vi "Get Analog Replay Settings.vi"(8 "error in (no error)":errorcluster, 11 "Analog Replay in":refnum<k24>) -> (0 "error out":errorcluster, 1 "Analog Replay Data Options":T1={"Input file"=path "", "Group"="", "Channel"="", "Reverse"=FALSE, "FPGA Memory Size"=enum."16,384", "Position reference"=enum."Crank angle", "Data selection method"=enum."Manual", "Offset"=0, "Samples"=0, "Missing teeth location"=0.0, "DataPlugin"=""}, 2 "Analog Replay Settings":T5={"Name"="", "DAC bipolar range (V)"=0.0, "Voltage below min speed"=0.0, "Min speed (RPM)"=0.0, "Voltage at min speed"=0.0, "Max speed (RPM)"=0.0, "Voltage at max speed"=0.0, "Negate playback voltage values at negative engine speed"=TRUE, "Allow run-time override of voltage scaling"=FALSE}, 3 "Analog Replay out":refnum<k24>)   [LabVIEW 2015, in "Engine Simulation Toolkit SysDef API.lvlib"]
uses:
  Engine Simulation Toolkit SysDef API.lvlib
  NationalInstruments.VeriStand.SystemDefinitionAPI
  Analog Replay Settings.ctl
  Analog Replay Data Options.ctl
  System Explorer/FPGA Mem Size.ctl
  System Explorer/Position Reference.ctl
  System Explorer/Data Replay Data Selection Method.ctl
  Shared/Properties.vi
  <vilib>/NI Veristand/Custom Device API/Get Item Property (String).vi
  <vilib>/NI Veristand/Custom Device API/Get Item Property (Double).vi
  <vilib>/NI Veristand/Custom Device API/Get Item Property (Boolean).vi
  Shared/Engine Simulation Toolkit Shared.lvlib
  System Explorer/Engine Simulation Toolkit System Explorer.lvlib
  <vilib>/NI VeriStand/Custom Device API/Custom Device API.lvlib
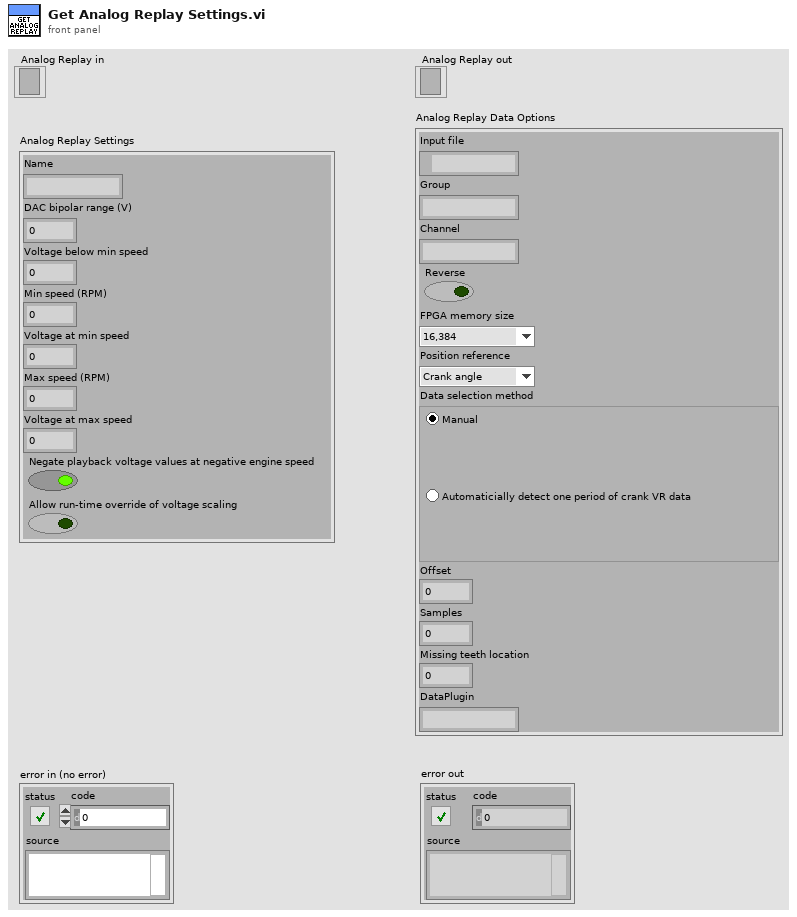
[diagram p1: front panel]
types:
  T1 = typedef "Engine Simulation Toolkit SysDef API.lvlib/Analog Replay Data Options.ctl" = cluster{"Input file":path, "Group":string, "Channel":string, "Reverse":bool, "FPGA Memory Size":T2, "Position reference":T3, "Data selection method":T4, "Offset":i32, "Samples":i32, "Missing teeth location":dbl, "DataPlugin":string}
  T2 = typedef "Engine Simulation Toolkit System Explorer.lvlib/FPGA Mem Size.ctl" = enum16{"65,536", "32,768", "16,384", "8,192", "4,096", "2,048", "1,024"}
  T3 = typedef "Engine Simulation Toolkit System Explorer.lvlib/Position Reference.ctl" = enum16{"Crank angle", "Cycle angle"}
  T4 = typedef "Engine Simulation Toolkit System Explorer.lvlib/Data Replay Data Selection Method.ctl" = enum32{"Manual", "AutoVRCrank"}
  T5 = typedef "Engine Simulation Toolkit SysDef API.lvlib/Analog Replay Settings.ctl" = cluster{"Name":string, "DAC bipolar range (V)":dbl, "Voltage below min speed":dbl, "Min speed (RPM)":dbl, "Voltage at min speed":dbl, "Max speed (RPM)":dbl, "Voltage at max speed":dbl, "Negate playback voltage values at negative engine speed":bool, "Allow run-time override of voltage scaling":bool}
  T6 = typedef "Custom Device API.lvlib/Custom Device Item Ref.ctl" = u64
  T7 = typedef "Engine Simulation Toolkit System Explorer.lvlib/File Load Dialog.ctl" = cluster{"File":path, "Group":string, "Channel":string, "DataPlugin":string, "MissingTeeth":dbl, "ErrState":string, "File Selected":bool, "Data Selection Method":T4, "Offset":i32, "Length":i32, "DataPlugins Info":T8[], "Controls":refnum<vi>[], "File Ref":refnum<k20>, "Groups":string[], "Channels":string[], "Groups Refs":refnum<k20>[], "Channel Refs":refnum<k20>[], "Cancelled":bool, "Position reference":T3, "FPGA memory size":T2, "GroupRef":refnum<k20>, "ChanRef":refnum<k20>, "Data":dbl[], "ReverseData":bool, "DispTwoRotations":bool, "cycle range":u16}
  T8 = typedef "usiPluginInformation.ctl" = cluster{"name":string, "version":string, "type":string, "read-only?":bool, "extensions":string[]}
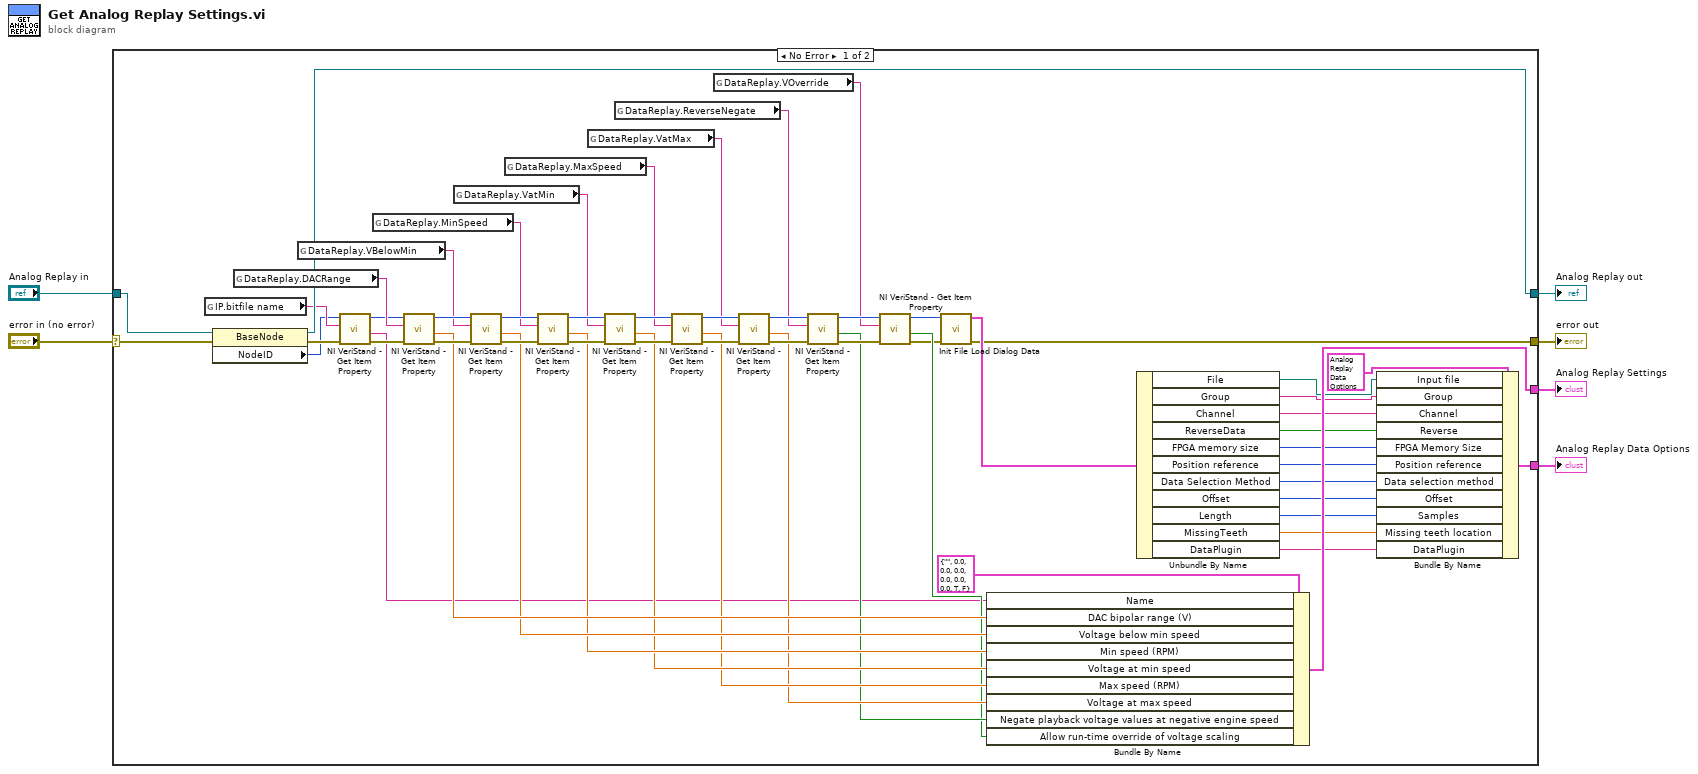
[diagram p0: block diagram]
diagram:
  n1 = case shown="No Error" "error in (no error)" {
    selector: "error in (no error)" -> [w13 w66]
    tunnel: "Analog Replay in" -> [w16 w65]
    tunnel: [w14 w65] -> w5
    tunnel: [w15 w66] -> w4
    tunnel: [w41 _] -> w3
    tunnel: [w39 _] -> w2
    frame No Error {
      n2 = global read "Properties.vi" "IP.bitfile name"() -> (w12:string)
      n3 = property class="BaseNode"(reference=w16, error in=w13) -> (reference out=w14:refnum<k24>, error out=w11:errorcluster, "NodeID"=w9:u64)
      n4 = global read "Properties.vi" "DataReplay.DACRange"() -> (w64:string)
      n5 = global read "Properties.vi" "DataReplay.VBelowMin"() -> (w61:string)
      n6 = call-poly <vilib>:"NI VeriStand - Get Item Property.vi"("error in (no error)"=w11, "Property Name"=w12, "Item Ref in"=w9) -> ("error out"=w10:errorcluster, "Value"=w7:string, "Item Ref out"=w8:T6)  [unwired: 5 in, 1 out]
      n7 = global read "Properties.vi" "DataReplay.MinSpeed"() -> (w54:string)
      n8 = call-poly <vilib>:"NI VeriStand - Get Item Property.vi"("error in (no error)"=w10, "Property Name"=w64, "Item Ref in"=w8) -> ("error out"=w62:errorcluster, "Value"=w38:dbl, "Item Ref out"=w63:T6)  [unwired: 5 in, 1 out]
      n9 = global read "Properties.vi" "DataReplay.VatMin"() -> (w51:string)
      n10 = call-poly <vilib>:"NI VeriStand - Get Item Property.vi"("error in (no error)"=w62, "Property Name"=w61, "Item Ref in"=w63) -> ("error out"=w55:errorcluster, "Value"=w37:dbl, "Item Ref out"=w56:T6)  [unwired: 5 in, 1 out]
      n11 = global read "Properties.vi" "DataReplay.MaxSpeed"() -> (w50:string)
      n12 = call-poly <vilib>:"NI VeriStand - Get Item Property.vi"("error in (no error)"=w55, "Property Name"=w54, "Item Ref in"=w56) -> ("error out"=w60:errorcluster, "Value"=w36:dbl, "Item Ref out"=w59:T6)  [unwired: 5 in, 1 out]
      n13 = global read "Properties.vi" "DataReplay.VatMax"() -> (w49:string)
      n14 = call-poly <vilib>:"NI VeriStand - Get Item Property.vi"("error in (no error)"=w60, "Property Name"=w51, "Item Ref in"=w59) -> ("error out"=w58:errorcluster, "Value"=w35:dbl, "Item Ref out"=w57:T6)  [unwired: 5 in, 1 out]
      n15 = global read "Properties.vi" "DataReplay.ReverseNegate"() -> (w44:string)
      n16 = call-poly <vilib>:"NI VeriStand - Get Item Property.vi"("error in (no error)"=w58, "Property Name"=w50, "Item Ref in"=w57) -> ("error out"=w53:errorcluster, "Value"=w34:dbl, "Item Ref out"=w52:T6)  [unwired: 5 in, 1 out]
      n17 = global read "Properties.vi" "DataReplay.VOverride"() -> (w43:string)
      n18 = call-poly <vilib>:"NI VeriStand - Get Item Property.vi"("error in (no error)"=w53, "Property Name"=w49, "Item Ref in"=w52) -> ("error out"=w48:errorcluster, "Value"=w33:dbl, "Item Ref out"=w47:T6)  [unwired: 5 in, 1 out]
      n19 = call-poly <vilib>:"NI VeriStand - Get Item Property.vi"("error in (no error)"=w48, "Property Name"=w44, "Item Ref in"=w47) -> ("error out"=w46:errorcluster, "Value"=w32:bool, "Item Ref out"=w45:T6)  [unwired: 5 in, 1 out]
      n20 = call-poly <vilib>:"NI VeriStand - Get Item Property.vi"("error in (no error)"=w46, "Property Name"=w43, "Item Ref in"=w45) -> ("error out"=w30:errorcluster, "Value"=w31:bool, "Item Ref out"=w29:T6)  [unwired: 5 in, 1 out]
      n21 = call "Init File Load Dialog Data.vi"("error in (no error)"=w30, "Node Ptr"=w29) -> ("error out"=w15:errorcluster, "FileDialog"=w28:T7)  [unwired: 8 in]
      n22 = Bundle By Name(cluster=T5 {"Name"="", "DAC bipolar range (V)"=0.0, "Voltage below min speed"=0.0, "Min speed (RPM)"=0.0, "Voltage at min speed"=0.0, "Max speed (RPM)"=0.0, "Voltage at max speed"=0.0, "Negate playback voltage values at negative engine speed"=TRUE, "Allow run-time override of voltage scaling"=FALSE} ("Analog Replay Settings"), "Name"=w7, "DAC bipolar range (V)"=w38, "Voltage below min speed"=w37, "Min speed (RPM)"=w36, "Voltage at min speed"=w35, "Max speed (RPM)"=w34, "Voltage at max speed"=w33, "Negate playback voltage values at negative engine speed"=w32, "Allow run-time override of voltage scaling"=w31) -> (w41:T5)
      n23 = Unbundle By Name(w28) -> ("File"=w27:path, "Group"=w26:string, "Channel"=w25:string, "ReverseData"=w24:bool, "FPGA memory size"=w23:T2, "Position reference"=w22:T3, "Data Selection Method"=w21:T4, "Offset"=w20:i32, "Length"=w19:i32, "MissingTeeth"=w18:dbl, "DataPlugin"=w17:string)
      n24 = Bundle By Name(cluster=T1 {"Input file"=path "", "Group"="", "Channel"="", "Reverse"=FALSE, "FPGA Memory Size"=enum."16,384", "Position reference"=enum."Crank angle", "Data selection method"=enum."Manual", "Offset"=0, "Samples"=0, "Missing teeth location"=0.0, "DataPlugin"=""} ("Analog Replay Data Options"), "Input file"=w27, "Group"=w26, "Channel"=w25, "Reverse"=w24, "FPGA Memory Size"=w23, "Position reference"=w22, "Data selection method"=w21, "Offset"=w20, "Samples"=w19, "Missing teeth location"=w18, "DataPlugin"=w17) -> (w39:T1)
    }
    frame Error {
    }
  }
  "Analog Replay out" <- w5
  "error out" <- w4
  "Analog Replay Settings" <- w3
  "Analog Replay Data Options" <- w2
